vi "Plotting XY Data with the Same X.vi"() -> ()   [LabVIEW 2012]
panel:
  in  "X Value":dbl format="%.1f"
  in  "stop":bool
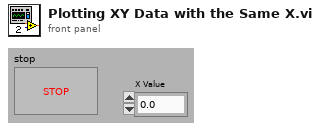
[diagram p1: front panel]
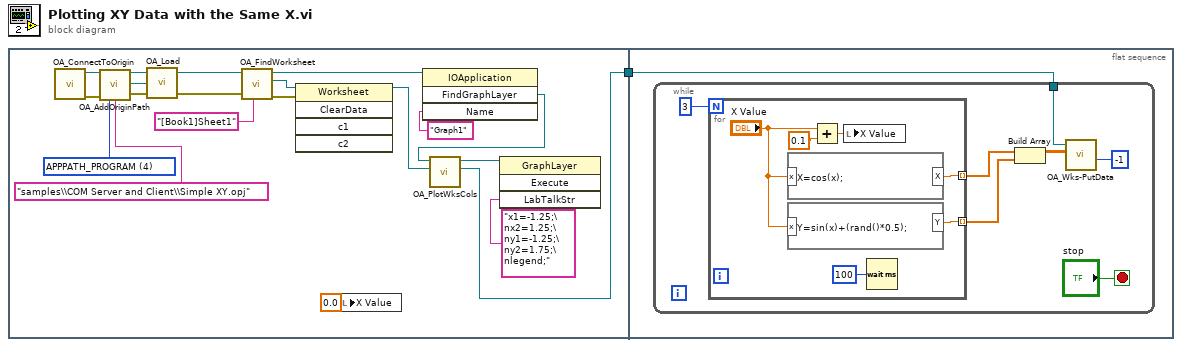
[diagram p0: block diagram]
diagram:
  n1 = flat-sequence {
    tunnel: [w2] -> w1
    tunnel: w1 -> [w22]
    frame #0 {
      w18 = 4 items=["APPPATH_USER"=2, "APPPATH_GROUP"=3, "APPPATH_PROGRAM"=4] ("Type")
      n2 = call "OA_ConnectToOrigin.vi"() -> ("error out"=w13:errorcluster, "Origin.IOApplication"=w20:refnum<k7>)  [unwired: 8 in]
      n3 = call "OA_AddOriginPath.vi"("Origin.IOApplication"=w20, "error in (no error)"=w13, "Type"=w18, "Filename"="samples\\COM Server and Client\\Simple XY.opj" ("related path")) -> ("Origin.IOApplication"=w15:refnum<k7>, "path out"=w17:path, "error out"=w16:errorcluster)  [unwired: 9 in]
      n4 = call "OA_Load.vi"("error in (no error)"=w16, "Path"=w17, "Origin.IOApplication"=w15) -> ("error out"=w10:errorcluster, "Origin.IOApplication"=w9:refnum<k7>)  [unwired: 1 out]
      n5 = call "OA_FindWorksheet.vi"("Name"="[Book1]Sheet1", "error in (no error)"=w10, "Origin.IOApplication"=w9) -> ("error out"=w11:errorcluster, "Origin.Worksheet"=w12:refnum<k7>, "Origin.IOApplication"=w7:refnum<k7>)  [unwired: 6 in]
      n6 = invoke class="Worksheet" method="ClearData"(reference=w12, error in=w11) -> (reference out=w6:refnum<k7>)  [unwired: 3 in, 4 out]
      n7 = local write "X Value"(0.0 ("X Value")) -> ()
      n8 = invoke class="IOApplication" method="FindGraphLayer"(reference=w7, "Name"="Graph1" ("related path")) -> ("FindGraphLayer"=w4:refnum<k7>)  [unwired: 2 in, 3 out]
      n9 = call "OA_PlotWksCols.vi"("Origin.Worksheet in"=w6, "Origin.GraphLayer in"=w4) -> ("Origin.Worksheet Out"=w2:refnum<k7>, "Origin.GraphLayer Out"=w3:refnum<k7>)  [unwired: 6 in, 2 out]
      n10 = invoke class="GraphLayer" method="Execute"(reference=w3, "LabTalkStr"="x1=-1.25;\nx2=1.25;\ny1=-1.25;\ny2=1.75;\nlegend;") -> ()  [unwired: 2 in, 4 out]
    }
    frame #1 {
      n11 = while {
        tunnel: w22 -> [w25]
        stop <- "stop" stop-if-true
        n12 = for {
          N: 3 -> [_]
          tunnel: [w35] -> w23 mode=indexing
          tunnel: [w31] -> w24 mode=indexing
          n13 = formula code="X=cos(x);"("x"="X Value") -> ("X"=w31:dbl)
          n14 = formula code="Y=sin(x)+(rand()*0.5);"("x"="X Value") -> ("Y"=w35:dbl)
          n15 = Add(x="X Value", y=0.1) -> (x+y=w32:dbl)
          n16 = local write "X Value"(w32) -> ()
          n17 = Wait (ms)(milliseconds to wait=u32 100) -> ()  [unwired: 1 out]
        }
        n18 = Build Array(w24, w23) -> (w28:dbl[][])
        n19 = call "OA_Wks-PutData.vi"("Row 1"=-1, "2d Data"=w28, "Origin.Worksheet"=w25) -> ()  [unwired: 2 in, 3 out]
      }
    }
  }
